vi "dnrm2 - Vector 2-Norm (DBL).vi"(7 "xInc":i32=1, 11 "x":dbl[](array[numeric])) -> (0 "error":i32, 3 "dnrm2":dbl)   [LabVIEW 2017, in "NI_AALBLAS.lvlib"]
doc: "Calculates the Euclidean norm of a vector."
uses:
  <vilib>/Analysis/NI_AALBLAS.lvlib
  <vilib>/Analysis/BLAS.llb/Fucntion.ctl
  <vilib>/Analysis/BLAS.llb/BLAS1 Utility(DBL).vi
panel:
  # "dnrm2=||x||"
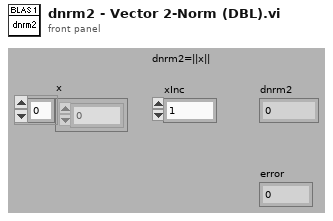
[diagram p1: front panel]
types:
  T1 = typedef "NI_AALBLAS.lvlib/Fucntion.ctl" = u16
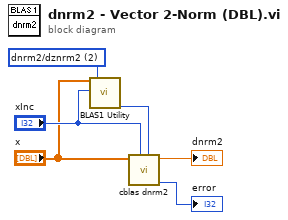
[diagram p0: block diagram]
diagram:
  w1 = T1 2 items=["ddot/zdotu/zdotc", "daxpy/zaxpy", "dnrm2/dznrm2", "dasum/dzasum", "dcopy/zcopy", "dswap/zswap", "drotm", "drot/zdrot", "idamax/izamax", "idamin/izamin", "dgemv/zgemv", "dsymv/zhemv", "dtrmv/ztrmv", "dsyr/zher", "dsyr2/zher2", "dger/zgeru/zgerc", "dtrsv/ztrsv", "dgemm/zgemm", "dsymm/zsymm/zhemm", "dtrmm/ztrmm", "dsyrk/zsyrk/zherk", "dsyr2k/zsyr2k/zher2k", "dtrsm/ztrsm"] ("function")
  n1 = call-poly <vilib>:"BLAS1 Utility.vi"("x"="x", "xInc"="xInc", "function"=w1) -> ("n"=w2:i32)  [unwired: 2 in, 14 out]
  n2 = call <vilib>:"cblas dnrm2.vi"("n"=w2, "incx"="xInc", "x"="x") -> ("error"=→"error":i32, "dnrm2"=→"dnrm2":dbl)  [unwired: 7 out]
